vi "testEmptyCount.vi"() -> (0 "error out":errorcluster)   [LabVIEW 2017, in "TestSuite.Tests.lvlib"]
uses:
  TestSuite.Tests.lvlib
  TestSuite/TestSuite.lvclass
  dbc93e30-74c4-4fe0-b447-585de9cc08e7.vi
  Constraint/IsEqual/Create.vi
  Constraint/IsEqual/IsEqual.lvclass
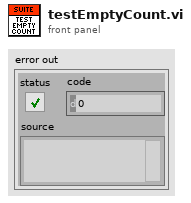
[diagram p1: front panel]
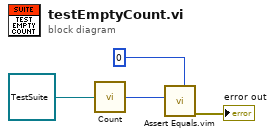
[diagram p0: block diagram]
diagram:
  n1 = call "Count.vi"("TestSuite In"=refnum<class "TestSuite.lvclass"> refnum ("TestSuite.lvclass")) -> ("Count"=w3:i32)
  n2 = call "Assert Equals.vim"("Expected"=0 ("Count"), "Actual"=w3) -> ("error out"=→"error out":errorcluster)  [unwired: 9 in]
